vi "SUP ps test.vi"() -> ()   [LabVIEW 2018]
panel:
  out "error out":errorcluster
  in  "Voltage":dbl=12.0
  in  "VISA name":refnum<visa-resource-name>="COM10"
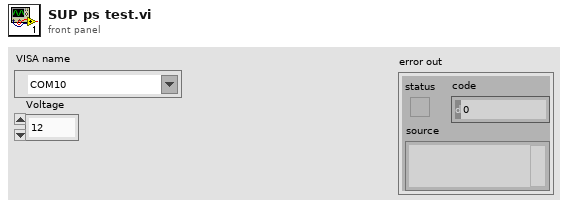
[diagram p1: front panel]
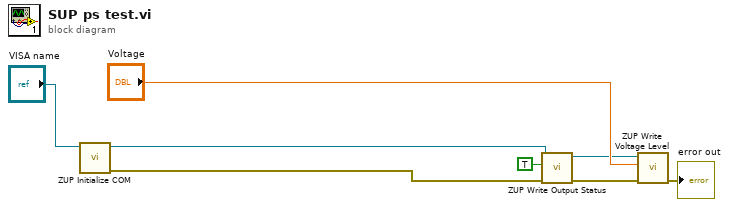
[diagram p0: block diagram]
diagram:
  n1 = call "ZUP Initialize COM.vi"("VISA resource name"="VISA name") -> ("error out"=w1:errorcluster, "VISA OUT"=w2:refnum<visa-resource-name>)  [unwired: 9 in]
  n2 = call "ZUP Write Output Status.vi"("error in (no error)"=w1, "ON/OFF"=TRUE, "VISA resource name"=w2) -> ("error out"=w5:errorcluster, "VISA OUT"=w6:refnum<visa-resource-name>)  [unwired: 6 in, 1 out]
  n3 = call "ZUP Write Voltage Level.vi"("error in (no error)"=w5, "Voltage"="Voltage", "VISA resource name"=w6) -> ("error out"=→"error out":errorcluster)  [unwired: 6 in, 2 out]
